vi "Get Acceleration.vi"(8 "error in (no error)":errorcluster, 11 "senseHatSensors in":refnum<class "RPI.SenseHat.Sensors.lvclass">) -> (0 "error out":errorcluster, 3 "senseHatSensors out":refnum<class "RPI.SenseHat.Sensors.lvclass">)   [LabVIEW 2020, in "RPI.SenseHat.Sensors.lvlib" / "RPI.SenseHat.Sensors.lvclass"]
uses:
  RPI.SenseHat.Sensors.lvclass
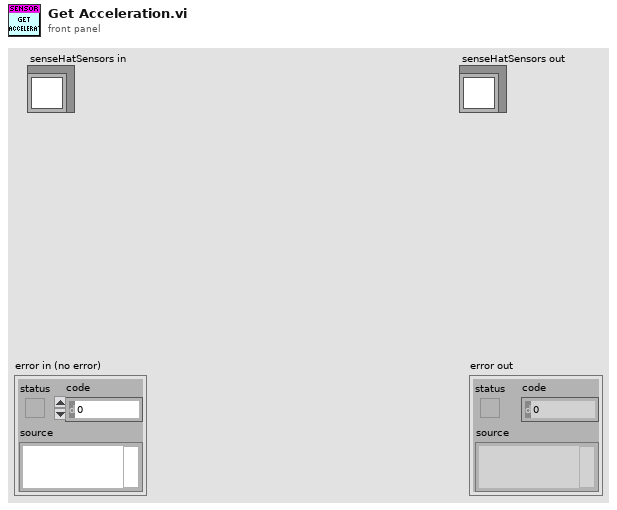
[diagram p1: front panel]
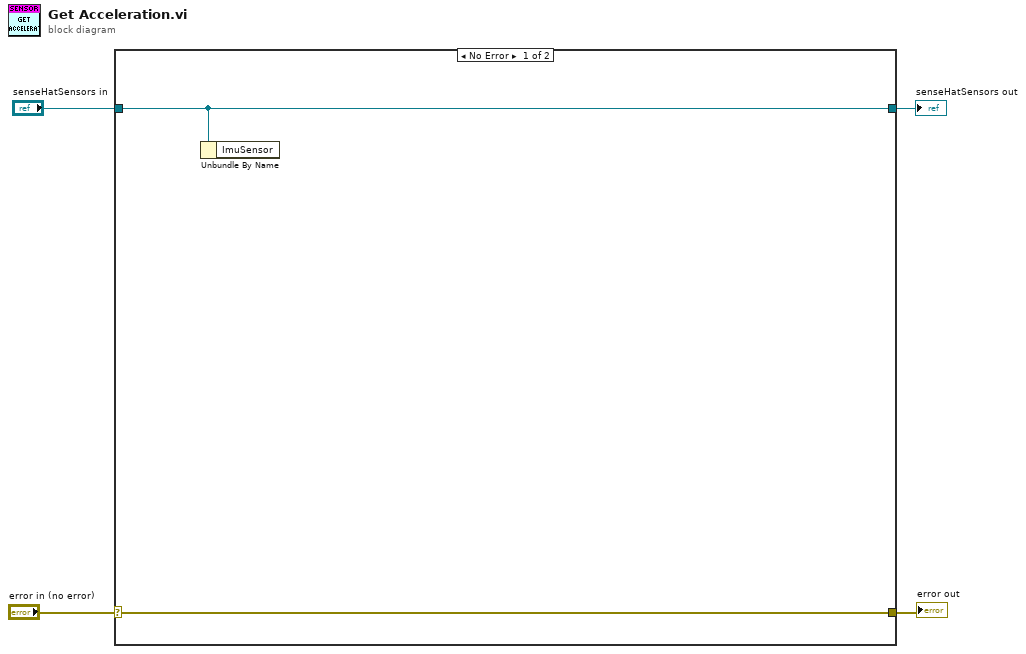
[diagram p0: block diagram]
diagram:
  n1 = case shown="No Error" "error in (no error)" {
    selector: "error in (no error)" -> [w6 w8]
    tunnel: [w6 w8] -> w3
    tunnel: [w5 w7] -> w1
    tunnel: "senseHatSensors in" -> [w5 w7]
    frame No Error {
      n2 = Unbundle By Name(w5) -> ()  [unwired: 1 out]
    }
    frame Error {
    }
  }
  "error out" <- w3
  "senseHatSensors out" <- w1
